vi "ex1.vi"() -> ()   [LabVIEW 2024]
panel:
  out "personne gauche":dbl(slide) scale=0.0..10.0
  out "personne droit":dbl(slide) scale=0.0..10.0
  out "rouge vers le droit":dbl(slide) scale=0.0..30.0
  out "noir decsendant":dbl(slide)
  out "bleu ascendant":dbl(slide) scale=0.0..30.0
  out "Rouge":bool
  out "vert":bool
  out "Rouge":bool
  out "orangè":bool
  out "vert":bool
  out "Rouge":bool
  out "vert":bool
  out "Rouge":bool
  out "orangè":bool
  out "vert":bool
  out "Rouge":bool
  out "vert":bool
  out "Rouge":bool
  out "orangè":bool
  out "vert":bool
  out "Rouge":bool
  out "vert":bool
  out "Rouge":bool
  out "orangè":bool
  out "vert":bool
  in  "Radio Buttons":enum32{"Mode Jour", "Mode Nuit"}(radio)
  out "orangè vers le gauche":dbl(slide)
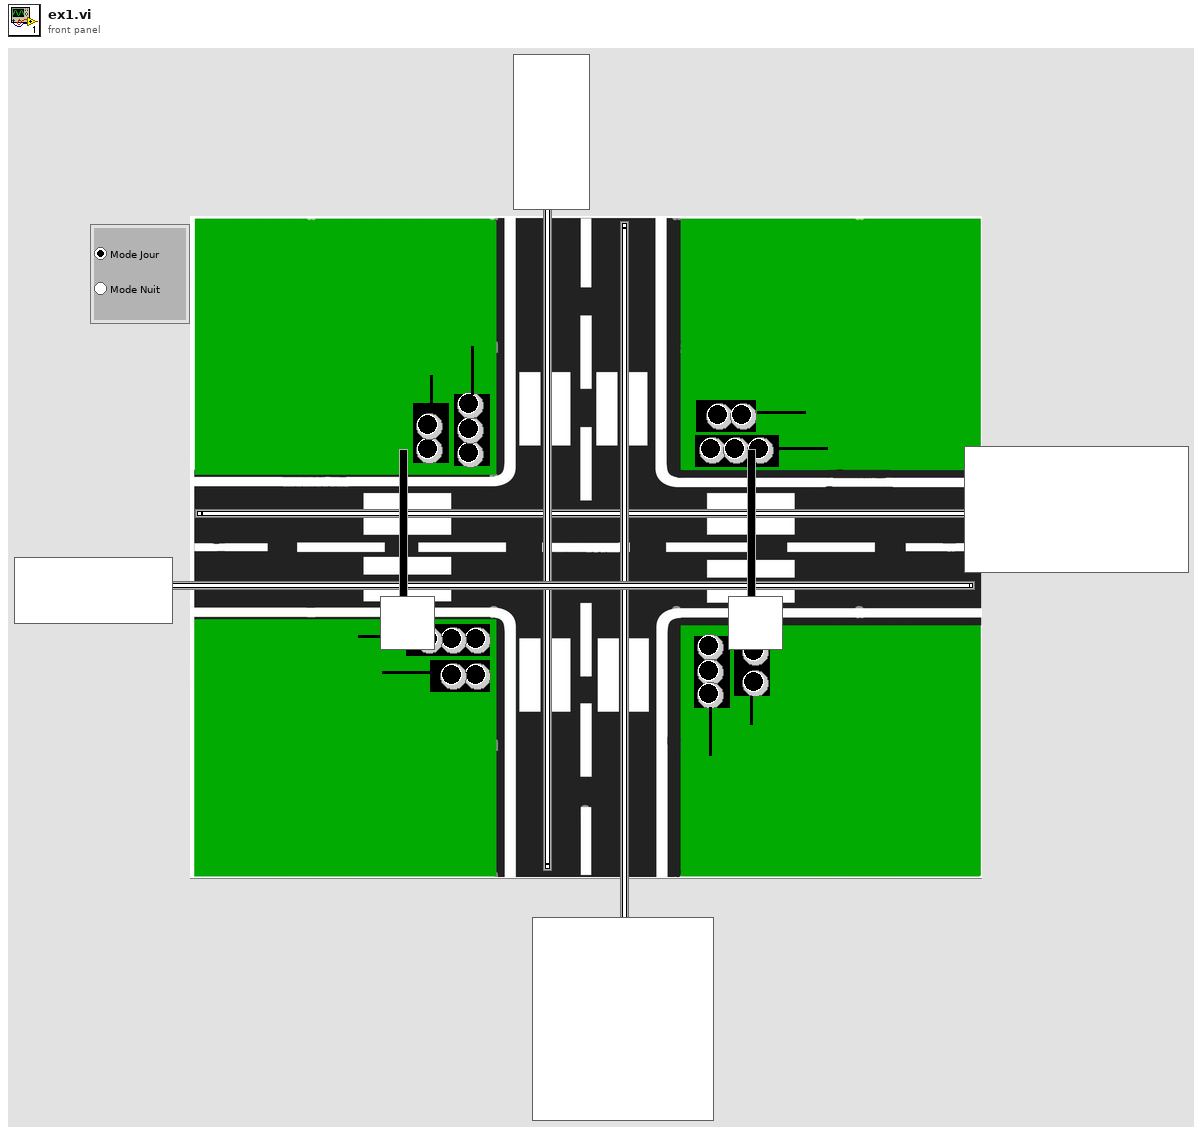
[diagram p1: front panel]
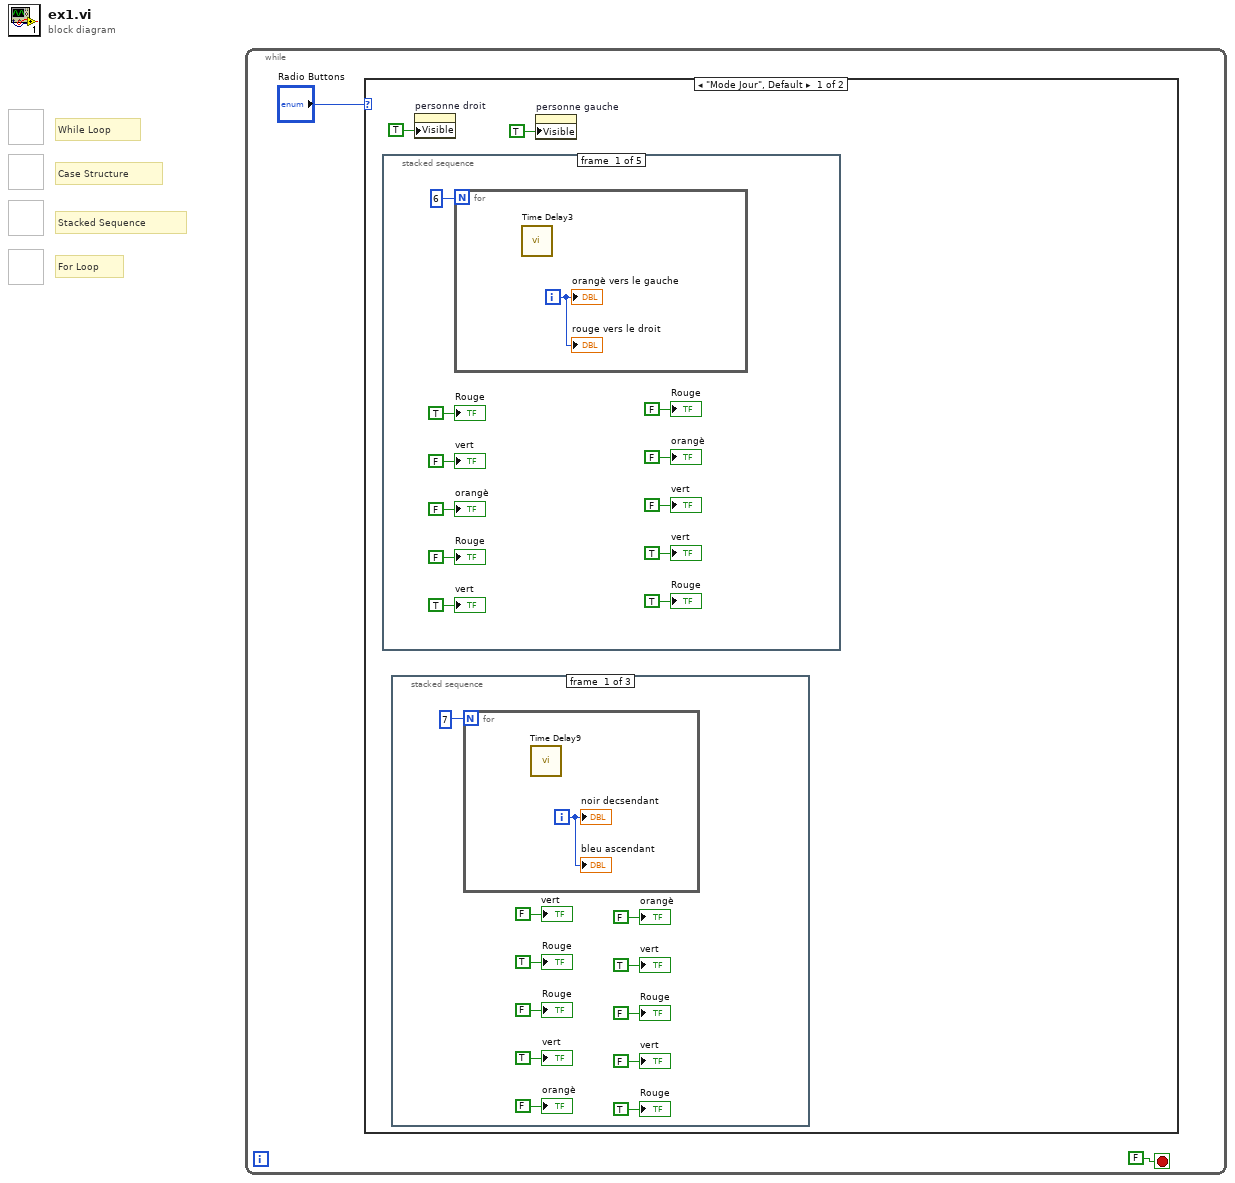
[diagram p0: block diagram]
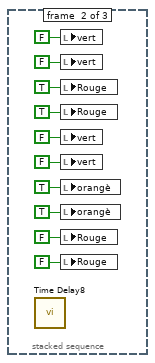
[diagram p2: hidden frame]
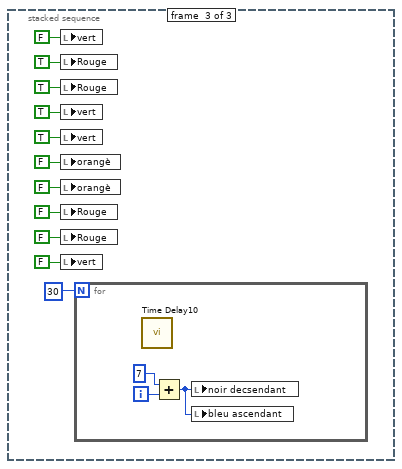
[diagram p3: hidden frame]
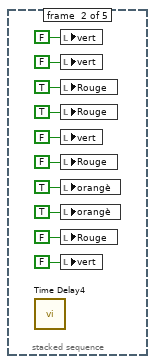
[diagram p4: hidden frame]
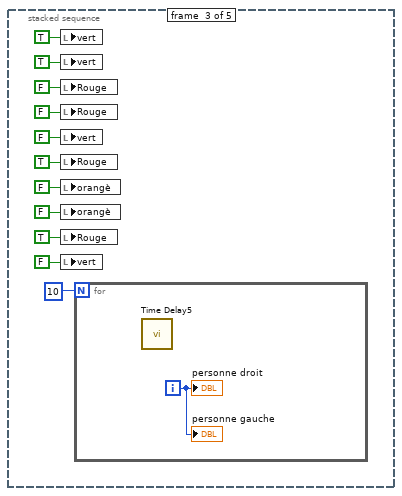
[diagram p5: hidden frame]
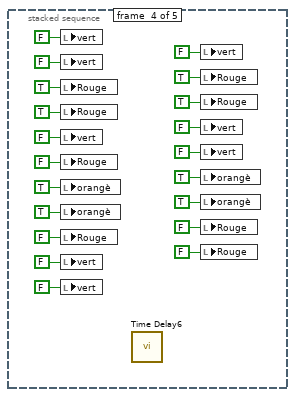
[diagram p6: hidden frame]
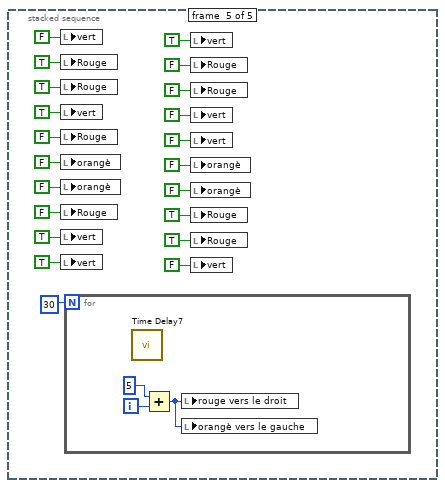
[diagram p7: hidden frame]
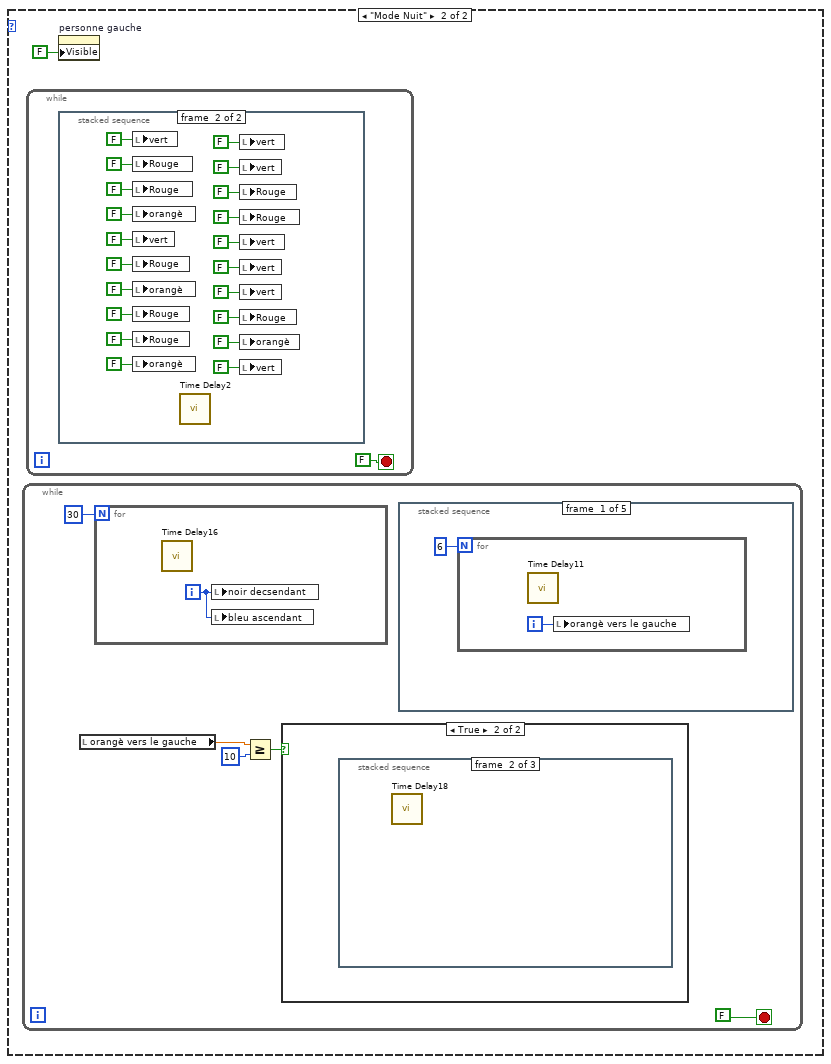
[diagram p8: hidden frame]
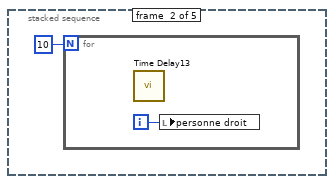
[diagram p9: hidden frame]
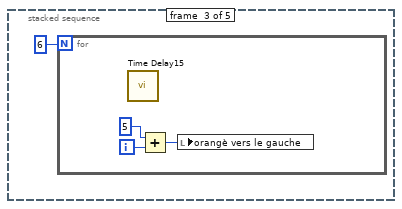
[diagram p10: hidden frame]
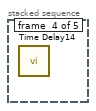
[diagram p11: hidden frame]
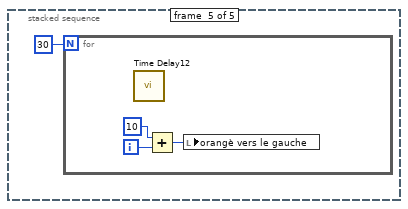
[diagram p12: hidden frame]
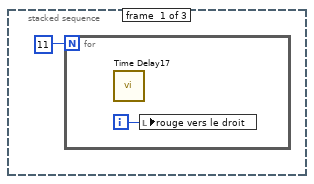
[diagram p14: hidden frame]
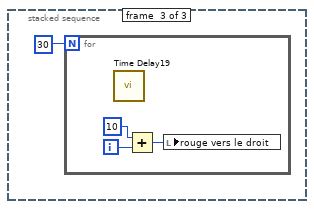
[diagram p15: hidden frame]
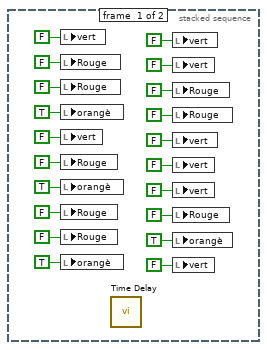
[diagram p16: hidden frame]
diagram:
  # "For Loop"
  # "Stacked Sequence"
  # "Case Structure"
  # "While Loop"
  n1 = while {
    stop <- FALSE stop-if-true
    n2 = case shown="\"Mode Jour\", Default" "Radio Buttons" {
      frame "Mode Jour", Default {
        n3 = stacked-sequence {
          frame #0 {
            n4 = for {
              N: 6 -> [_]
              i -> [w52]
              n5 = call "Time Delay3"() -> ()  [unwired: 11 in, 1 out]
              "orangè vers le gauche" <- w52
              "rouge vers le droit" <- w52
            }
            "Rouge" <- FALSE ("Rouge")
            "orangè" <- FALSE ("orangè")
            "vert" <- TRUE ("vert")
            "Rouge" <- TRUE ("Rouge")
            "vert" <- FALSE ("vert")
            "vert" <- TRUE ("vert")
            "orangè" <- FALSE ("orangè")
            "Rouge" <- FALSE ("Rouge")
            "Rouge" <- TRUE ("Rouge")
            "vert" <- FALSE ("vert")
          }
          frame #1 {
            n6 = call "Time Delay4"() -> ()  [unwired: 11 in, 1 out]
            n7 = local write "vert"(FALSE ("vert")) -> ()
            n8 = local write "vert"(FALSE ("vert")) -> ()
            n9 = local write "Rouge"(TRUE ("Rouge")) -> ()
            n10 = local write "Rouge"(TRUE ("Rouge")) -> ()
            n11 = local write "vert"(FALSE ("vert")) -> ()
            n12 = local write "Rouge"(FALSE ("Rouge")) -> ()
            n13 = local write "orangè"(TRUE ("orangè")) -> ()
            n14 = local write "orangè"(TRUE ("orangè")) -> ()
            n15 = local write "Rouge"(FALSE ("Rouge")) -> ()
            n16 = local write "vert"(FALSE ("vert")) -> ()
          }
          frame #2 {
            n17 = local write "vert"(TRUE ("vert")) -> ()
            n18 = local write "vert"(TRUE ("vert")) -> ()
            n19 = local write "Rouge"(FALSE ("Rouge")) -> ()
            n20 = local write "Rouge"(FALSE ("Rouge")) -> ()
            n21 = local write "vert"(FALSE ("vert")) -> ()
            n22 = local write "Rouge"(TRUE ("Rouge")) -> ()
            n23 = local write "orangè"(FALSE ("orangè")) -> ()
            n24 = local write "orangè"(FALSE ("orangè")) -> ()
            n25 = local write "Rouge"(TRUE ("Rouge")) -> ()
            n26 = local write "vert"(FALSE ("vert")) -> ()
            n27 = for {
              N: 10 -> [_]
              i -> [w74]
              n28 = call "Time Delay5"() -> ()  [unwired: 11 in, 1 out]
              "personne gauche" <- w74
              "personne droit" <- w74
            }
          }
          frame #3 {
            n29 = local write "vert"(FALSE ("vert")) -> ()
            n30 = local write "vert"(FALSE ("vert")) -> ()
            n31 = local write "Rouge"(TRUE ("Rouge")) -> ()
            n32 = local write "Rouge"(TRUE ("Rouge")) -> ()
            n33 = local write "vert"(FALSE ("vert")) -> ()
            n34 = local write "Rouge"(FALSE ("Rouge")) -> ()
            n35 = local write "orangè"(TRUE ("orangè")) -> ()
            n36 = local write "orangè"(TRUE ("orangè")) -> ()
            n37 = local write "Rouge"(FALSE ("Rouge")) -> ()
            n38 = local write "vert"(FALSE ("vert")) -> ()
            n39 = local write "vert"(FALSE ("vert")) -> ()
            n40 = call "Time Delay6"() -> ()  [unwired: 11 in, 1 out]
            n41 = local write "vert"(FALSE ("vert")) -> ()
            n42 = local write "Rouge"(TRUE ("Rouge")) -> ()
            n43 = local write "Rouge"(TRUE ("Rouge")) -> ()
            n44 = local write "vert"(FALSE ("vert")) -> ()
            n45 = local write "vert"(FALSE ("vert")) -> ()
            n46 = local write "orangè"(TRUE ("orangè")) -> ()
            n47 = local write "orangè"(TRUE ("orangè")) -> ()
            n48 = local write "Rouge"(FALSE ("Rouge")) -> ()
            n49 = local write "Rouge"(FALSE ("Rouge")) -> ()
          }
          frame #4 {
            n50 = local write "vert"(FALSE ("vert")) -> ()
            n51 = local write "Rouge"(TRUE ("Rouge")) -> ()
            n52 = local write "Rouge"(TRUE ("Rouge")) -> ()
            n53 = local write "vert"(TRUE ("vert")) -> ()
            n54 = local write "Rouge"(FALSE ("Rouge")) -> ()
            n55 = local write "orangè"(FALSE ("orangè")) -> ()
            n56 = local write "orangè"(FALSE ("orangè")) -> ()
            n57 = local write "Rouge"(FALSE ("Rouge")) -> ()
            n58 = local write "vert"(TRUE ("vert")) -> ()
            n59 = local write "vert"(TRUE ("vert")) -> ()
            n60 = for {
              N: 30 -> [_]
              i -> [w118]
              n61 = call "Time Delay7"() -> ()  [unwired: 11 in, 1 out]
              n62 = Add(x=5, y=w118) -> (x+y=w116:i32)
              n63 = local write "rouge vers le droit"(w116) -> ()
              n64 = local write "orangè vers le gauche"(w116) -> ()
            }
            n65 = local write "vert"(TRUE ("vert")) -> ()
            n66 = local write "Rouge"(FALSE ("Rouge")) -> ()
            n67 = local write "Rouge"(FALSE ("Rouge")) -> ()
            n68 = local write "vert"(FALSE ("vert")) -> ()
            n69 = local write "vert"(FALSE ("vert")) -> ()
            n70 = local write "orangè"(FALSE ("orangè")) -> ()
            n71 = local write "orangè"(FALSE ("orangè")) -> ()
            n72 = local write "Rouge"(TRUE ("Rouge")) -> ()
            n73 = local write "Rouge"(TRUE ("Rouge")) -> ()
            n74 = local write "vert"(FALSE ("vert")) -> ()
          }
        }
        n75 = stacked-sequence {
          frame #0 {
            n76 = for {
              N: 7 -> [_]
              i -> [w16]
              n77 = call "Time Delay9"() -> ()  [unwired: 11 in, 1 out]
              "noir decsendant" <- w16
              "bleu ascendant" <- w16
            }
            "Rouge" <- TRUE ("Rouge")
            "orangè" <- FALSE ("orangè")
            "vert" <- FALSE ("vert")
            "Rouge" <- FALSE ("Rouge")
            "vert" <- TRUE ("vert")
            "Rouge" <- TRUE ("Rouge")
            "orangè" <- FALSE ("orangè")
            "vert" <- FALSE ("vert")
            "Rouge" <- FALSE ("Rouge")
            "vert" <- TRUE ("vert")
          }
          frame #1 {
            n78 = call "Time Delay8"() -> ()  [unwired: 11 in, 1 out]
            n79 = local write "vert"(FALSE ("vert")) -> ()
            n80 = local write "vert"(FALSE ("vert")) -> ()
            n81 = local write "Rouge"(TRUE ("Rouge")) -> ()
            n82 = local write "Rouge"(TRUE ("Rouge")) -> ()
            n83 = local write "vert"(FALSE ("vert")) -> ()
            n84 = local write "vert"(FALSE ("vert")) -> ()
            n85 = local write "orangè"(TRUE ("orangè")) -> ()
            n86 = local write "orangè"(TRUE ("orangè")) -> ()
            n87 = local write "Rouge"(FALSE ("Rouge")) -> ()
            n88 = local write "Rouge"(FALSE ("Rouge")) -> ()
          }
          frame #2 {
            n89 = local write "vert"(FALSE ("vert")) -> ()
            n90 = local write "Rouge"(TRUE ("Rouge")) -> ()
            n91 = local write "Rouge"(TRUE ("Rouge")) -> ()
            n92 = local write "vert"(TRUE ("vert")) -> ()
            n93 = local write "vert"(TRUE ("vert")) -> ()
            n94 = local write "orangè"(FALSE ("orangè")) -> ()
            n95 = local write "orangè"(FALSE ("orangè")) -> ()
            n96 = local write "Rouge"(FALSE ("Rouge")) -> ()
            n97 = local write "Rouge"(FALSE ("Rouge")) -> ()
            n98 = local write "vert"(FALSE ("vert")) -> ()
            n99 = for {
              N: 30 -> [_]
              i -> [w39]
              n100 = call "Time Delay10"() -> ()  [unwired: 11 in, 1 out]
              n101 = Add(x=7, y=w39) -> (x+y=w38:i32)
              n102 = local write "noir decsendant"(w38) -> ()
              n103 = local write "bleu ascendant"(w38) -> ()
            }
          }
        }
        n104 = property on="personne droit" class="Slide (strict)"("Visible"=TRUE) -> ()  [unwired: 2 in, 2 out]
        n105 = property on="personne gauche" class="Slide (strict)"("Visible"=TRUE) -> ()  [unwired: 2 in, 2 out]
      }
      frame "Mode Nuit" {
        n106 = while {
          stop <- FALSE stop-if-true
          n107 = local read "orangè vers le gauche"() -> (w122:dbl)
          n108 = for {
            N: 30 -> [_]
            i -> [w143]
            n109 = call "Time Delay16"() -> ()  [unwired: 11 in, 1 out]
            n110 = local write "noir decsendant"(w143) -> ()
            n111 = local write "bleu ascendant"(w143) -> ()
          }
          n112 = Greater Or Equal?(x=w122, y=10) -> (x >= y?=w123:bool)
          n113 = case shown="True" w123 {
            frame False {
            }
            frame True {
              n114 = stacked-sequence {
                frame #0 {
                  n115 = for {
                    N: 11 -> [_]
                    i -> [w138]
                    n116 = call "Time Delay17"() -> ()  [unwired: 11 in, 1 out]
                    n117 = local write "rouge vers le droit"(w138) -> ()
                  }
                }
                frame #1 {
                  n118 = call "Time Delay18"() -> ()  [unwired: 11 in, 1 out]
                }
                frame #2 {
                  n119 = for {
                    N: 30 -> [_]
                    i -> [w141]
                    n120 = call "Time Delay19"() -> ()  [unwired: 11 in, 1 out]
                    n121 = Add(x=10, y=w141) -> (x+y=w140:i32)
                    n122 = local write "rouge vers le droit"(w140) -> ()
                  }
                }
              }
            }
          }
          n123 = stacked-sequence {
            frame #0 {
              n124 = for {
                N: 6 -> [_]
                i -> [w126]
                n125 = call "Time Delay11"() -> ()  [unwired: 11 in, 1 out]
                n126 = local write "orangè vers le gauche"(w126) -> ()
              }
            }
            frame #1 {
              n127 = for {
                N: 10 -> [_]
                i -> [w128]
                n128 = call "Time Delay13"() -> ()  [unwired: 11 in, 1 out]
                n129 = local write "personne droit"(w128) -> ()
              }
            }
            frame #2 {
              n130 = for {
                N: 6 -> [_]
                i -> [w130]
                n131 = call "Time Delay15"() -> ()  [unwired: 11 in, 1 out]
                n132 = Add(x=5, y=w130) -> (x+y=w131:i32)
                n133 = local write "orangè vers le gauche"(w131) -> ()
              }
            }
            frame #3 {
              n134 = call "Time Delay14"() -> ()  [unwired: 11 in, 1 out]
            }
            frame #4 {
              n135 = for {
                N: 30 -> [_]
                i -> [w135]
                n136 = call "Time Delay12"() -> ()  [unwired: 11 in, 1 out]
                n137 = Add(x=10, y=w135) -> (x+y=w134:i32)
                n138 = local write "orangè vers le gauche"(w134) -> ()
              }
            }
          }
        }
        n139 = while {
          stop <- FALSE stop-if-true
          n140 = stacked-sequence {
            frame #0 {
              n141 = local write "vert"(FALSE ("vert")) -> ()
              n142 = local write "Rouge"(FALSE ("Rouge")) -> ()
              n143 = local write "Rouge"(FALSE ("Rouge")) -> ()
              n144 = local write "orangè"(TRUE ("orangè")) -> ()
              n145 = local write "vert"(FALSE ("vert")) -> ()
              n146 = local write "Rouge"(FALSE ("Rouge")) -> ()
              n147 = local write "orangè"(TRUE ("orangè")) -> ()
              n148 = local write "Rouge"(FALSE ("Rouge")) -> ()
              n149 = local write "Rouge"(FALSE ("Rouge")) -> ()
              n150 = local write "orangè"(TRUE ("orangè")) -> ()
              n151 = call "Time Delay"() -> ()  [unwired: 11 in, 1 out]
              n152 = local write "vert"(FALSE ("vert")) -> ()
              n153 = local write "vert"(FALSE ("vert")) -> ()
              n154 = local write "Rouge"(FALSE ("Rouge")) -> ()
              n155 = local write "Rouge"(FALSE ("Rouge")) -> ()
              n156 = local write "vert"(FALSE ("vert")) -> ()
              n157 = local write "vert"(FALSE ("vert")) -> ()
              n158 = local write "vert"(FALSE ("vert")) -> ()
              n159 = local write "Rouge"(FALSE ("Rouge")) -> ()
              n160 = local write "orangè"(TRUE ("orangè")) -> ()
              n161 = local write "vert"(FALSE ("vert")) -> ()
            }
            frame #1 {
              n162 = local write "vert"(FALSE ("vert")) -> ()
              n163 = local write "Rouge"(FALSE ("Rouge")) -> ()
              n164 = local write "Rouge"(FALSE ("Rouge")) -> ()
              n165 = local write "orangè"(FALSE ("orangè")) -> ()
              n166 = local write "vert"(FALSE ("vert")) -> ()
              n167 = local write "Rouge"(FALSE ("Rouge")) -> ()
              n168 = local write "orangè"(FALSE ("orangè")) -> ()
              n169 = local write "Rouge"(FALSE ("Rouge")) -> ()
              n170 = local write "Rouge"(FALSE ("Rouge")) -> ()
              n171 = local write "orangè"(FALSE ("orangè")) -> ()
              n172 = call "Time Delay2"() -> ()  [unwired: 11 in, 1 out]
              n173 = local write "vert"(FALSE ("vert")) -> ()
              n174 = local write "vert"(FALSE ("vert")) -> ()
              n175 = local write "Rouge"(FALSE ("Rouge")) -> ()
              n176 = local write "Rouge"(FALSE ("Rouge")) -> ()
              n177 = local write "vert"(FALSE ("vert")) -> ()
              n178 = local write "vert"(FALSE ("vert")) -> ()
              n179 = local write "vert"(FALSE ("vert")) -> ()
              n180 = local write "Rouge"(FALSE ("Rouge")) -> ()
              n181 = local write "orangè"(FALSE ("orangè")) -> ()
              n182 = local write "vert"(FALSE ("vert")) -> ()
            }
          }
        }
        n183 = property on="personne gauche" class="Slide (strict)"("Visible"=FALSE) -> ()  [unwired: 2 in, 2 out]
      }
    }
  }
